vi "Sort Modules.vi"(8 "error in (no error)":errorcluster, 10 "Modules":refnum<class "Module.lvclass">[](array[class]), 11 "Block Diagram in":refnum<class "Block Diagram.lvclass">) -> (0 "error out":errorcluster, 3 "Block Diagram out":refnum<class "Block Diagram.lvclass">)   [LabVIEW 2015, in "Block Diagram.lvclass"]
uses:
  Block Diagram.lvclass
  Module/Module Class/Module.lvclass
  Block Diagram.lvclass/Block Diagram.ctl
  Module Loop/Module Loop.lvclass
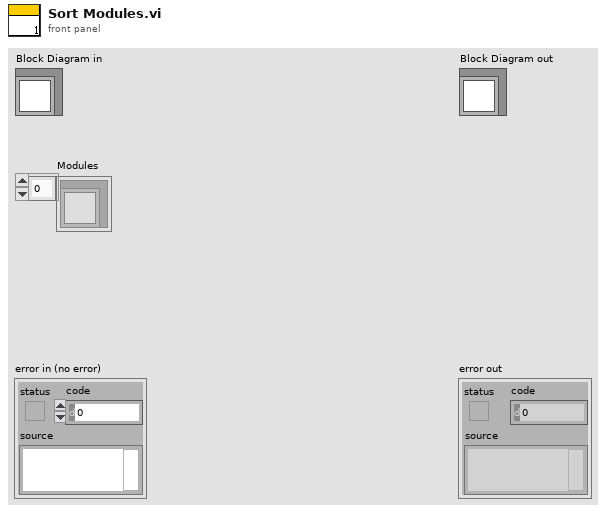
[diagram p1: front panel]
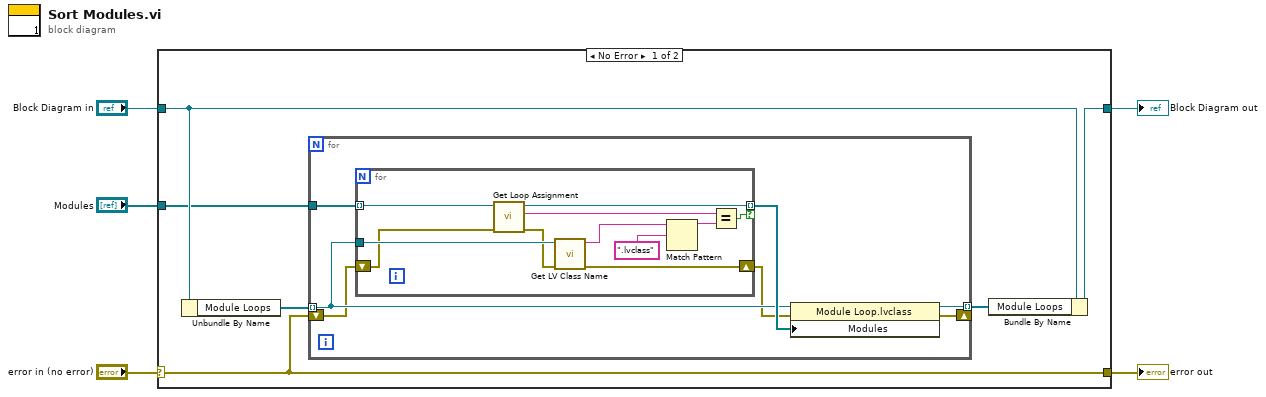
[diagram p0: block diagram]
diagram:
  n1 = case shown="No Error" "error in (no error)" {
    selector: "error in (no error)" -> [w10 w31]
    tunnel: [w10 w31] -> w4
    tunnel: [w11 w30] -> w2
    tunnel: "Block Diagram in" -> [w9 w30]
    tunnel: "Modules" -> [w6 _]
    frame No Error {
      n2 = Unbundle By Name(w9) -> ("Module Loops"=w8:refnum<class "Module Loop.lvclass">[])
      n3 = for {
        tunnel: w6 -> [w18]
        tunnel: w8 -> [w16] mode=indexing
        tunnel: [w15] -> w7 mode=indexing
        shift-right: [w13] -> _
        shift-left: w10 -> [w12]
        n4 = for {
          tunnel: w18 -> [w19] mode=indexing
          tunnel: w16 -> [w29]
          tunnel: [w23] -> w17 mode=indexing if=w22
          shift-right: [w21] -> w14
          shift-left: w12 -> [w20]
          n5 = call "Get Loop Assignment.vi"("error in (no error)"=w20, "Module in"=w19) -> ("error out"=w28:errorcluster, "Loop Assignment"=w24:string, "Module out"=w23:refnum<class "Module.lvclass">)  [unwired: 7 in]
          n6 = call <vilib>:"Get LV Class Name.vi"("error in (no error)"=w28, "object"=w29) -> ("error out"=w21:errorcluster, "class name"=w27:string)  [unwired: 8 in]
          n7 = Match Pattern(string=w27, regular expression=".lvclass") -> (before substring=w25:string)  [unwired: 1 in, 3 out]
          n8 = Equal?(x=w24, y=w25) -> (x = y?=w22:bool)
        }
        n9 = property class="Module Loop.lvclass"(reference=w16, error in=w14, "Modules"=w17) -> (reference out=w15:refnum<class "Module Loop.lvclass">, error out=w13:errorcluster)
      }
      n10 = Bundle By Name(cluster=w9, "Module Loops"=w7) -> (w11:refnum<class "Block Diagram.lvclass">)
    }
    frame Error {
    }
  }
  "error out" <- w4
  "Block Diagram out" <- w2
